vi "stop.vi"(8 "error in":errorcluster, 11 "Basic HTTP server in":refnum<class "Basic HTTP server.lvclass">) -> (0 "error out":errorcluster)   [LabVIEW 2016, in "Basic HTTP server.lvclass"]
uses:
  Basic HTTP server.lvclass
  Basic HTTP server.lvclass/Basic HTTP server.ctl
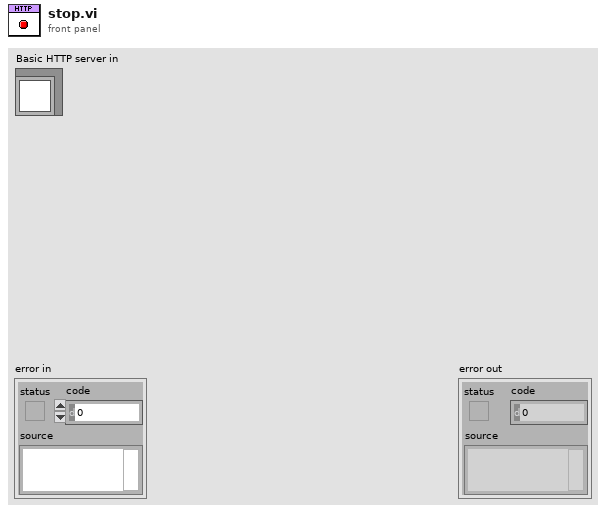
[diagram p1: front panel]
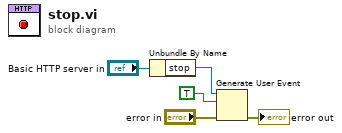
[diagram p0: block diagram]
diagram:
  n1 = Unbundle By Name("Basic HTTP server in") -> ("stop"=w2:refnum<user-event>)
  n2 = Generate User Event(user event=w2, event data cluster=TRUE ("event data"), error in="error in") -> (error out=→"error out":errorcluster)  [unwired: 1 in, 1 out]
